vi "Update In World.vi"(11 "Asteroid in":refnum<class "Asteroid.lvclass">) -> (3 "Asteroid out":refnum<class "Asteroid.lvclass">)   [LabVIEW 2021, in "Asteroid.lvclass"]
uses:
  Asteroid.lvclass
  C:/dev/LabVIEW/LabMelee/Source/Application Specific/Element/Element.lvclass
  Asteroid.lvclass/Asteroid.ctl
  Element/Element.lvclass
  <userlib>/_OpenG.lib/numeric/numeric.llb/openg_numeric__ogtk.lvlib
  <userlib>/_OpenG.lib/numeric/numeric.llb/Random Number Within Range - DBL__ogtk.vi
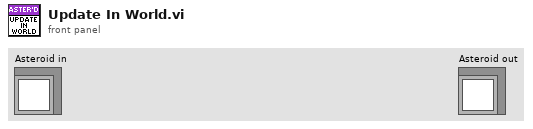
[diagram p1: front panel]
types:
  T1 = typedef "Constants.ctl" = cluster{"Colours":cluster{"OK":u32, "Warning":u32, "Error":u32, "Red":u32, "Green":u32, "Blue":u32, "Yellow":u32}, "System":cluster{"Target Frames Second":dbl, "World Size":T2, "Window Size":T2, "Viewport Size":T2, "Sidebar Scaling":sgl, "Sidebar Width":i32, "SC2 Frame Rate [Seconds/Frame]":sgl}, "Game":cluster{"Maximum Asteroids":i32, "Max Energy":i32, "Max Crew":i32, "Maximum Stars":i32}}
  T2 = typedef "SDL2 Utility.lvlib/Point (I32).ctl" = cluster{"x":i32, "y":i32}
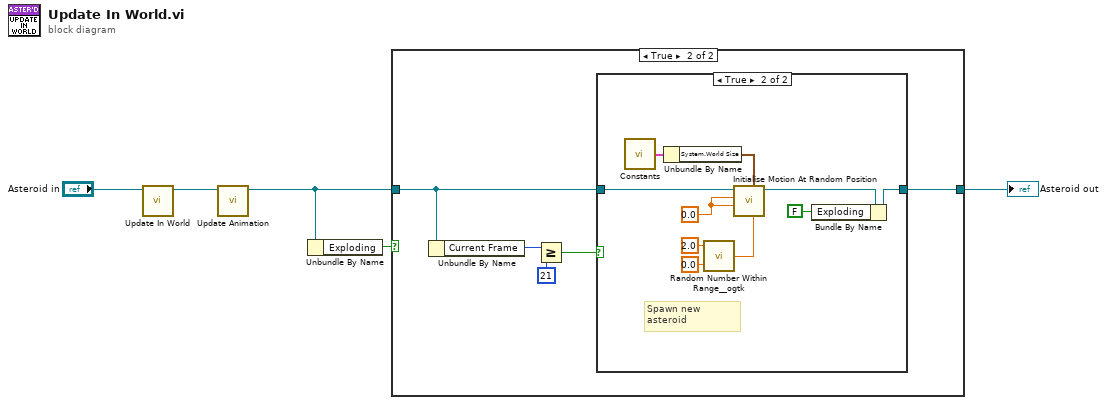
[diagram p0: block diagram]
diagram:
  n1 = call-parent "Update In World.vi"("Movable in"="Asteroid in") -> ("Movable out"=w4:refnum<class "Asteroid.lvclass">)  [unwired: 10 in]
  n2 = call "Update Animation.vi"("Asteroid in"=w4) -> ("Asteroid out"=w2:refnum<class "Asteroid.lvclass">)  [unwired: 10 in]
  n3 = Unbundle By Name(w2) -> ("Exploding"=w3:bool)
  n4 = case shown="True" w3 {
    tunnel: [w6 w8] -> w1
    tunnel: w2 -> [w6 w11]
    frame False {
    }
    frame True {
      n5 = Unbundle By Name(w11) -> ("Current Frame"=w7:i32)
      n6 = Greater Or Equal?(x=w7, y=21) -> (x >= y?=w9:bool)
      n7 = case shown="True" w9 {
        tunnel: [w12 w14] -> w8
        tunnel: w11 -> [w12 w22]
        frame False {
        }
        frame True {
          w21 = sgl 0.0 ("Turn Rate [deg/s]")
          # "Spawn new asteroid"
          n8 = call "Constants.vi"() -> ("Constants"=w20:T1)
          n9 = Unbundle By Name(w20) -> ("System.World Size"=w19:T2)
          n10 = call-poly <userlib>:"Random Number Within Range__ogtk.vi"("High"=sgl 2.0 ("Initial Heading [deg]"), "Low"=sgl 0.0 ("Initial Heading [deg]")) -> ("Random Number"=w16:dbl)  [unwired: 3 in]
          n11 = call "Initialise Motion At Random Position.vi"("Initial Velocity [m/s]"=w16, "Field Size"=w19, "Acceleration [m/s/s]"=w21, "Turn Rate [deg/s]"=w21, "Movable in"=w22) -> ("Movable out"=w15:refnum<class "Asteroid.lvclass">)  [unwired: 6 in]
          n12 = Bundle By Name(cluster=w15, "Exploding"=FALSE) -> (w14:refnum<class "Asteroid.lvclass">)
        }
      }
    }
  }
  "Asteroid out" <- w1
